vi "currentTime.vi"() -> (5 "Hour":i32, 6 "Minute":i32, 7 "Second":i32)   [LabVIEW 2013]
doc: "VI gets current system time and outputs Hour Minute and Second as 2 digit integer"
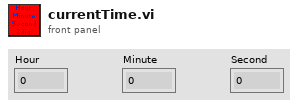
[diagram p1: front panel]
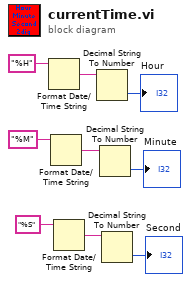
[diagram p0: block diagram]
diagram:
  n1 = Format Date/Time String(time format string (%c)="%H") -> (date/time string=w6:string)  [unwired: 2 in]
  n2 = Format Date/Time String(time format string (%c)="%M") -> (date/time string=w5:string)  [unwired: 2 in]
  n3 = Format Date/Time String(time format string (%c)="%S") -> (date/time string=w4:string)  [unwired: 2 in]
  n4 = Decimal String To Number(string=w6) -> (number=→"Hour":i32)  [unwired: 2 in, 1 out]
  n5 = Decimal String To Number(string=w5) -> (number=→"Minute":i32)  [unwired: 2 in, 1 out]
  n6 = Decimal String To Number(string=w4) -> (number=→"Second":i32)  [unwired: 2 in, 1 out]
